vi "Handle Controller.vi"(7 "Processing In":refnum<class "Processing.lvclass">, 10 "Controller in":refnum<class "Controller.lvclass">, 11 "Arguments Handler in":refnum<class "ControllerIndexedPathParams Handler.lvclass">) -> (0 "error out":errorcluster, 2 "Controller":refnum<class "Controller.lvclass">, 5 "Processing":refnum<class "Processing.lvclass">)   [LabVIEW 2020, in "HTTP Server.lvlib" / "ControllerIndexedPathParams Handler.lvclass"]
uses:
  ControllerIndexedPathParams Handler.lvclass
  ControllerIndexedPathParams Handler.lvclass/ControllerIndexedPathParams Handler.ctl
  Processing/Processing.lvclass
  Values/Values.lvclass
  lv-uri/URI/URI.lvlib
  Controller/Controller.lvclass
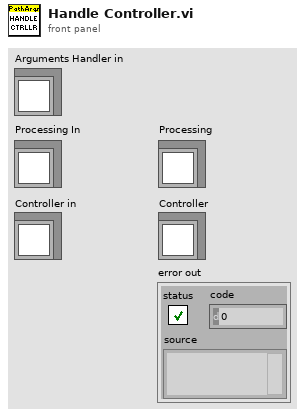
[diagram p1: front panel]
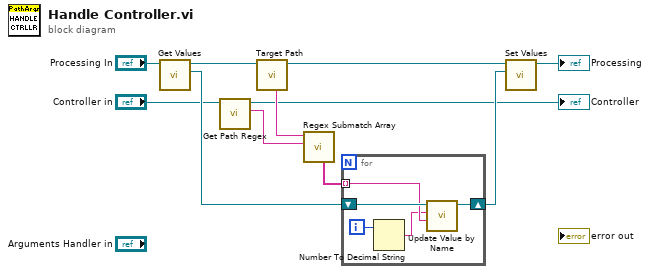
[diagram p0: block diagram]
diagram:
  n1 = call "Get Values.vi"("Processing in"="Processing In") -> ("Values"=w5:refnum<class "Values.lvclass">, "Processing out"=w2:refnum<class "Processing.lvclass">)  [unwired: 9 in]
  n2 = call-dynamic "Get Path Regex.vi"("Controller in"="Controller in") -> ("Path Regex"=w11:string, "Controller out"=→"Controller":refnum<class "Controller.lvclass">)  [unwired: 8 in, 1 out]
  n3 = call "Target Path.vi"("Processing in"=w2) -> ("Processing out"=w8:refnum<class "Processing.lvclass">, "Target Path"=w9:string)  [unwired: 9 in]
  n4 = call "Regex Submatch Array.vi"("regular expression"=w11, "string"=w9) -> ("matches"=w10:string[])  [unwired: 5 in, 4 out]
  n5 = for {
    shift-right: [w14] -> w7
    shift-left: w5 -> [w15]
    tunnel: w10 -> [w13] mode=indexing
    i -> [w16]
    n6 = Number To Decimal String(number=w16) -> (decimal integer string=w12:string)  [unwired: 1 in]
    n7 = call "Update Value by Name.vi"("Value"=w13, "Name"=w12, "Values in"=w15) -> ("Values out"=w14:refnum<class "Values.lvclass">)  [unwired: 7 in, 1 out]
  }
  n8 = call "Set Values.vi"("Values"=w7, "Processing in"=w8) -> ("Processing out"=→"Processing":refnum<class "Processing.lvclass">)  [unwired: 9 in]
